vi "Double to Fixed-Point Raw Data.vi"(8 "isSigned?":bool=TRUE, 9 "data":dbl format="%#_13g", 10 "delta":dbl format="%#_13g", 11 "word length":i8) -> (3 "Value":i64)   [LabVIEW 2018]
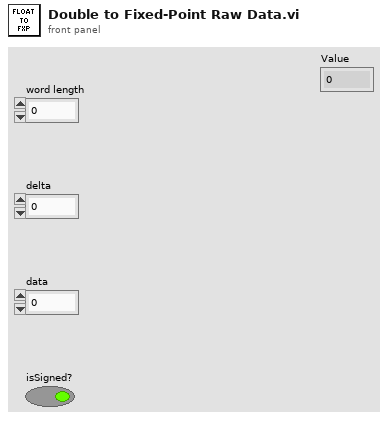
[diagram p1: front panel]
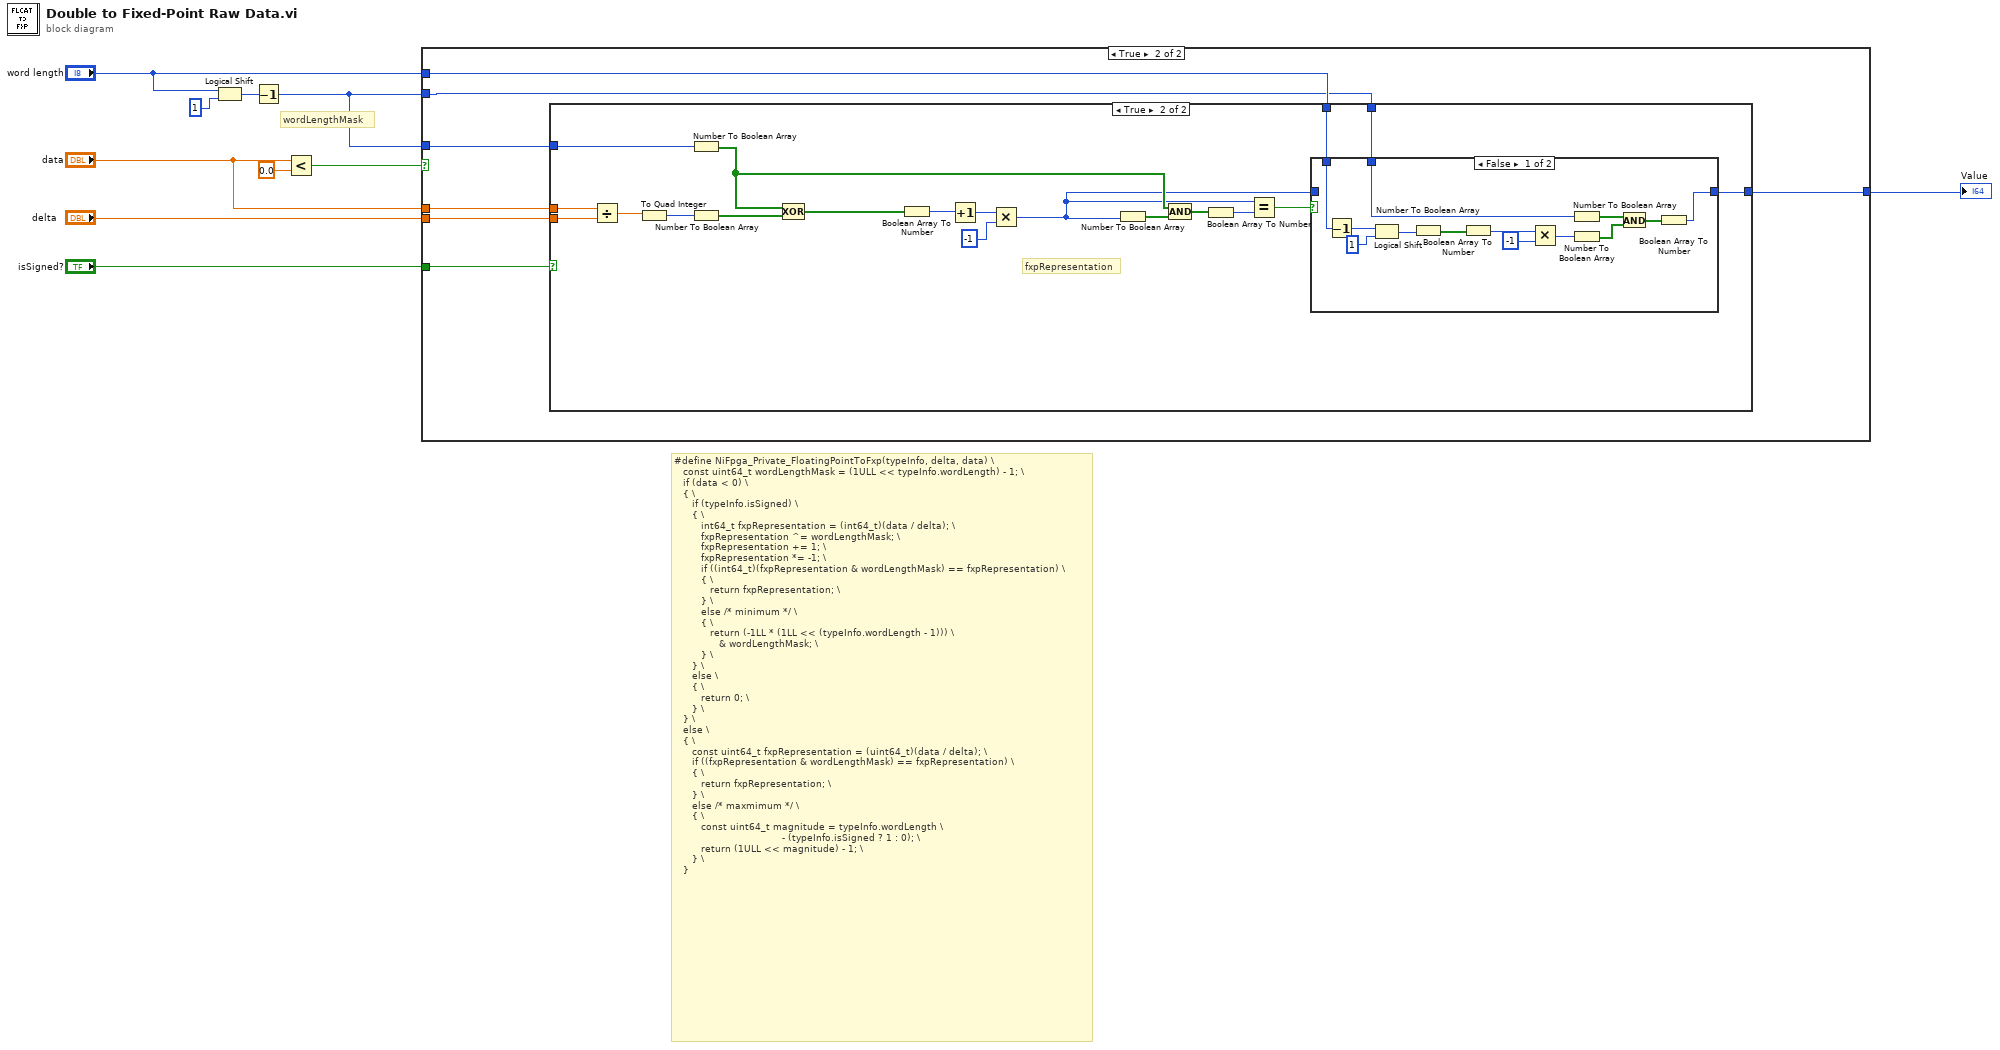
[diagram p0: block diagram]
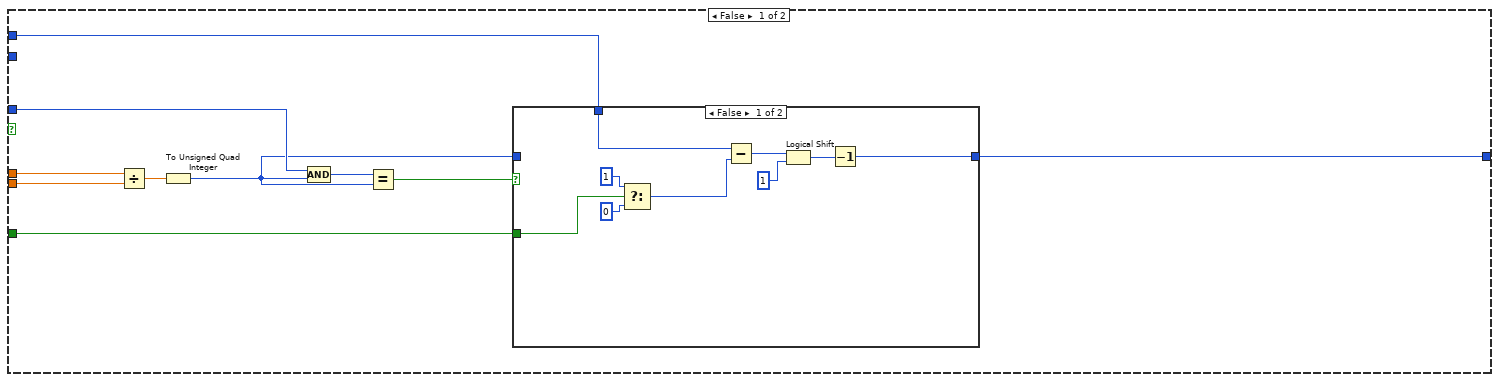
[diagram p2: hidden frame]
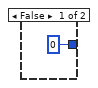
[diagram p4: hidden frame]
diagram:
  # "wordLengthMask"
  # "#define NiFpga_Private_FloatingPointToFxp(typeInfo, delta, data) \\\n   const uint64_t wordLengthMask = (1ULL << typeInfo.wordLength) - 1; \\\n   if (data < 0) \\\n   { \\\n      if (typeInfo.isSigned) \\\n      { \\\n         int64_t fxpRepresentation = (int64_t)(data / delta); \\\n         fxpRepresentation ^= wordLengthMask; \\\n         fxpRepresentation += 1; \\\n         fxpRepresentation *= -1; \\\n         if ((int64_t)(fxpRepresentation & wordLengthMask) == fxpRepresentation) \\\n         { \\\n            return fxpRepresentation; \\\n         } \\\n         else /* minimum */ \\\n         { \\\n            return (-1LL * (1LL << (typeInfo.wordLength - 1))) \\\n               & wordLengthMask; \\\n         } \\\n      } \\\n      else \\\n      { \\\n         return 0; \\\n      } \\\n   } \\\n   else \\\n   { \\\n      const uint64_t fxpRepresentation = (uint64_t)(data / delta); \\\n      if ((fxpRepresentation & wordLengthMask) == fxpRepresentation) \\\n      { \\\n         return fxpRepresentation; \\\n      } \\\n      else /* maxmimum */ \\\n      { \\\n         const uint64_t magnitude = typeInfo.wordLength \\\n                                    - (typeInfo.isSigned ? 1 : 0); \\\n         return (1ULL << magnitude) - 1; \\\n      } \\\n   }"
  n1 = Logical Shift(y="word length", x=u64 1) -> (x << y=w10:u64)
  n2 = Decrement(x=w10) -> (x-1=w1:u64)
  n3 = Less?(x="data", y=0.0) -> (x < y?=w7:bool)
  n4 = case shown="True" w7 {
    tunnel: "isSigned?" -> [w11 w37]
    tunnel: "data" -> [w20 w36]
    tunnel: "delta" -> [w19 w35]
    tunnel: w1 -> [w17 w34]
    tunnel: [w13 w33] -> w3
    tunnel: "word length" -> [w12 w32]
    tunnel: w1 -> [_ w31]
    frame False {
      n5 = Divide(x=w20, y=w19) -> (x/y=w18:dbl)
      n6 = To Unsigned Quad Integer(1:w18) -> (0:w14:u64)
      n7 = Compound Arithmetic op=AND(w17, w14) -> (w16:u64)
      n8 = Equal?(x=w16, y=w14) -> (x = y?=w15:bool)
      n9 = case shown="False" w15 {
        tunnel: w14 -> [_ w30]
        tunnel: [w21 w30] -> w13
        tunnel: w12 -> [w26 _]
        tunnel: w11 -> [w29 _]
        frame False {
          n10 = Select(t=u8 1 ("word length"), s=w29, f=u8 0) -> (s? t:f=w25:u8)
          n11 = Subtract(x=w26, y=w25) -> (x-y=w24:u8)
          n12 = Logical Shift(y=w24, x=u64 1) -> (x << y=w22:u64)
          n13 = Decrement(x=w22) -> (x-1=w21:u64)
        }
        frame True {
        }
      }
    }
    frame True {
      n14 = case shown="True" w37 {
        tunnel: w36 -> [_ w57]
        tunnel: w35 -> [_ w56]
        tunnel: w34 -> [_ w54]
        tunnel: [i64 0 w41] -> w33
        tunnel: w32 -> [_ w40]
        tunnel: w31 -> [_ w39]
        frame False {
        }
        frame True {
          # "fxpRepresentation"
          n15 = Divide(x=w57, y=w56) -> (x/y=w55:dbl)
          n16 = To Quad Integer(1:w55) -> (0:w53:i64)
          n17 = Number To Boolean Array(number=w54) -> (Boolean array=w47:bool[])
          n18 = Number To Boolean Array(number=w53) -> (Boolean array=w52:bool[])
          n19 = Compound Arithmetic op=XOR(w47, w52) -> (w51:bool[])
          n20 = Boolean Array To Number(Boolean array=w51) -> (number=w50:i64)
          n21 = Increment(x=w50) -> (x+1=w49:i64)
          n22 = Multiply(x=w49, y=i64 -1) -> (x*y=w42:i64)
          n23 = Number To Boolean Array(number=w42) -> (Boolean array=w46:bool[])
          n24 = Compound Arithmetic op=AND(w47, w46) -> (w45:bool[])
          n25 = Boolean Array To Number(Boolean array=w45) -> (number=w44:i64)
          n26 = Equal?(x=w42, y=w44) -> (x = y?=w43:bool)
          n27 = case shown="False" w43 {
            tunnel: w42 -> [_ w71]
            tunnel: [w58 w71] -> w41
            tunnel: w40 -> [w68 _]
            tunnel: w39 -> [w62 _]
            frame False {
              n28 = Decrement(x=w68) -> (x-1=w69:i8)
              n29 = Logical Shift(y=w69, x=u64 1) -> (x << y=w67:u64)
              n30 = Number To Boolean Array(number=w67) -> (Boolean array=w66:bool[])
              n31 = Boolean Array To Number(Boolean array=w66) -> (number=w65:i64)
              n32 = Multiply(x=w65, y=i64 -1) -> (x*y=w63:i64)
              n33 = Number To Boolean Array(number=w62) -> (Boolean array=w61:bool[])
              n34 = Number To Boolean Array(number=w63) -> (Boolean array=w60:bool[])
              n35 = Compound Arithmetic op=AND(w61, w60) -> (w59:bool[])
              n36 = Boolean Array To Number(Boolean array=w59) -> (number=w58:i64)
            }
            frame True {
            }
          }
        }
      }
    }
  }
  "Value" <- w3
